vi "SW_Smooth_Image.vi"(6 "Normalize? (F)":bool, 7 "Sigma":dbl=1.0, 8 "Error In":errorcluster, 9 "Image? (T)":bool=TRUE, 10 "Array or pixmap in":u32[][](array[numeric]), 11 "Kernel size":u32=5) -> (0 "Error Out":errorcluster, 3 "Array or pixmap out":u32[][](array[numeric]))   [LabVIEW 2018, in "Tracker.lvlib"]
uses:
  Tracker.lvlib
  <vilib>/Analysis/2dsp.llb/2D Convolution (DBL).vi
  <vilib>/Analysis/NI_AALPro.lvlib
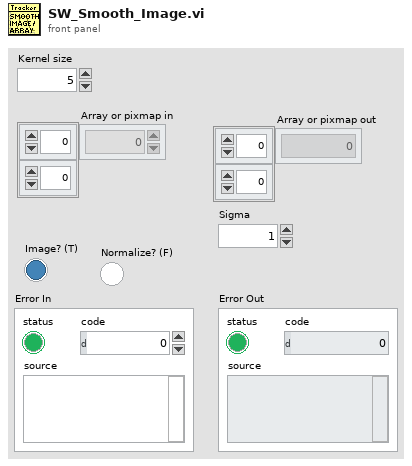
[diagram p1: front panel]
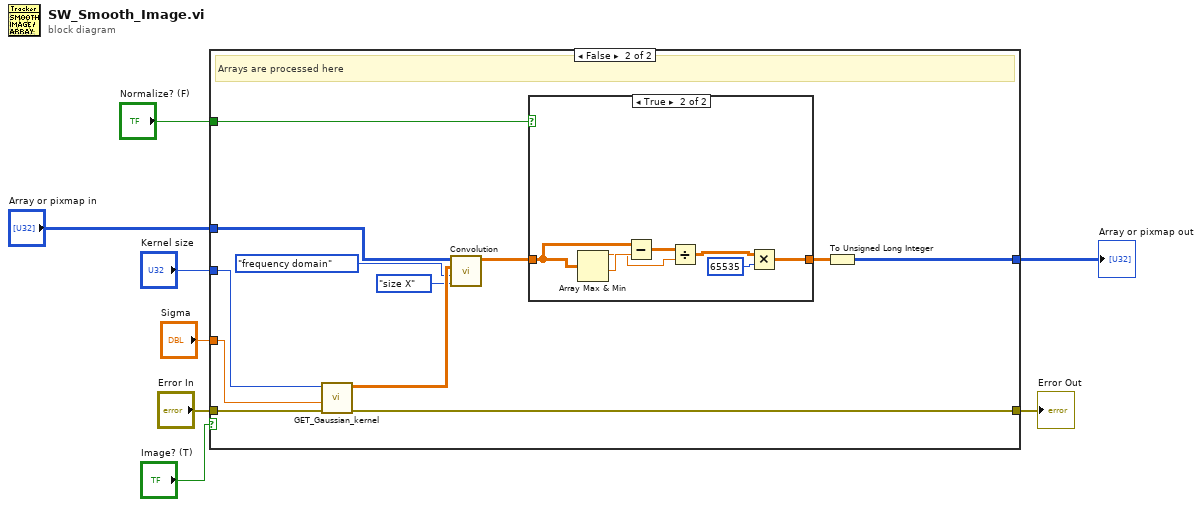
[diagram p0: block diagram]
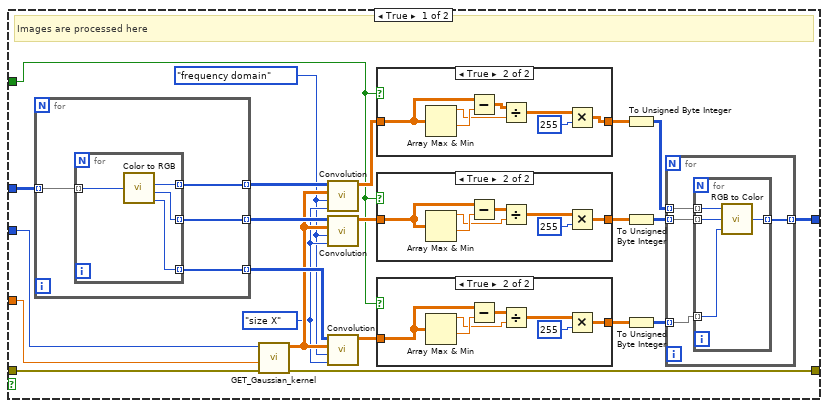
[diagram p2: hidden frame]
diagram:
  n1 = case shown="False" "Image? (T)" {
    tunnel: "Array or pixmap in" -> [w30 w77]
    tunnel: "Kernel size" -> [w29 w82]
    tunnel: "Sigma" -> [w28 w81]
    tunnel: [w18 w74] -> w4
    tunnel: "Error In" -> [w17 w76]
    tunnel: [w16 w75] -> w2
    tunnel: "Normalize? (F)" -> [w10 w71]
    frame True {
      w23 = enum32{"full", "size X", "compact"}."size X" ("output size")
      w22 = enum32{"direct", "frequency domain"}."frequency domain" ("algorithm")
      # "Images are processed here"
      n2 = for {
        tunnel: w30 -> [w66] mode=indexing
        tunnel: [w65] -> w27 mode=indexing
        tunnel: [w64] -> w26 mode=indexing
        tunnel: [w63] -> w25 mode=indexing
        n3 = for {
          tunnel: w66 -> [w70] mode=indexing
          tunnel: [w69] -> w65 mode=indexing
          tunnel: [w68] -> w64 mode=indexing
          tunnel: [w67] -> w63 mode=indexing
          n4 = call <vilib>:"Color to RGB.vi"("Color"=w70) -> ("R"=w69:u8, "G"=w68:u8, "B"=w67:u8)  [unwired: 1 out]
        }
      }
      n5 = call "GET_Gaussian_kernel.vi"("Error In"=w17, "Sigma"=w28, "Kernel size"=w29) -> ("Error Out"=w16:errorcluster, "Gaussian kernel (normalized)"=w24:dbl[][])  [unwired: 7 in]
      n6 = call-poly <vilib>:"Convolution.vi"("output size"=w23, "algorithm"=w22, "Y"=w24, "X"=w27) -> ("X * Y"=w15:dbl[][])  [unwired: 6 in, 1 out]
      n7 = call-poly <vilib>:"Convolution.vi"("output size"=w23, "algorithm"=w22, "Y"=w24, "X"=w26) -> ("X * Y"=w13:dbl[][])  [unwired: 6 in, 1 out]
      n8 = call-poly <vilib>:"Convolution.vi"("output size"=w23, "algorithm"=w22, "Y"=w24, "X"=w25) -> ("X * Y"=w11:dbl[][])  [unwired: 6 in, 1 out]
      n9 = case shown="True" w10 {
        tunnel: w15 -> [w47 w54]
        tunnel: [w47 w48] -> w14
        frame False {
        }
        frame True {
          n10 = Array Max & Min(array=w54) -> (max value=w51:dbl, min value=w53:dbl)  [unwired: 2 out]
          n11 = Subtract(x=w54, y=w53) -> (x-y=w52:dbl[][])
          n12 = Divide(x=w52, y=w51) -> (x/y=w50:dbl[][])
          n13 = Multiply(x=w50, y=255) -> (x*y=w48:dbl[][])
        }
      }
      n14 = case shown="True" w10 {
        tunnel: w13 -> [w39 w46]
        tunnel: [w39 w40] -> w12
        frame False {
        }
        frame True {
          n15 = Array Max & Min(array=w46) -> (max value=w43:dbl, min value=w45:dbl)  [unwired: 2 out]
          n16 = Subtract(x=w46, y=w45) -> (x-y=w44:dbl[][])
          n17 = Divide(x=w44, y=w43) -> (x/y=w42:dbl[][])
          n18 = Multiply(x=w42, y=255) -> (x*y=w40:dbl[][])
        }
      }
      n19 = case shown="True" w10 {
        tunnel: w11 -> [w31 w38]
        tunnel: [w31 w32] -> w9
        frame False {
        }
        frame True {
          n20 = Array Max & Min(array=w38) -> (max value=w35:dbl, min value=w37:dbl)  [unwired: 2 out]
          n21 = Subtract(x=w38, y=w37) -> (x-y=w36:dbl[][])
          n22 = Divide(x=w36, y=w35) -> (x/y=w34:dbl[][])
          n23 = Multiply(x=w34, y=255) -> (x*y=w32:dbl[][])
        }
      }
      n24 = To Unsigned Byte Integer(number=w14) -> (unsigned 8bit integer=w21:u8[][])
      n25 = To Unsigned Byte Integer(number=w12) -> (unsigned 8bit integer=w20:u8[][])
      n26 = To Unsigned Byte Integer(number=w9) -> (unsigned 8bit integer=w19:u8[][])
      n27 = for {
        tunnel: w21 -> [w58] mode=indexing
        tunnel: w20 -> [w57] mode=indexing
        tunnel: w19 -> [w56] mode=indexing
        tunnel: [w55] -> w18 mode=indexing
        n28 = for {
          tunnel: w58 -> [w62] mode=indexing
          tunnel: w57 -> [w61] mode=indexing
          tunnel: w56 -> [w60] mode=indexing
          tunnel: [w59] -> w55 mode=indexing
          n29 = call <vilib>:"RGB to Color.vi"("B"=w60, "G"=w61, "R"=w62) -> ("Color"=w59:u32)
        }
      }
    }
    frame False {
      # "Arrays are processed here"
      n30 = call "GET_Gaussian_kernel.vi"("Error In"=w76, "Sigma"=w81, "Kernel size"=w82) -> ("Error Out"=w75:errorcluster, "Gaussian kernel (normalized)"=w80:dbl[][])  [unwired: 7 in]
      n31 = call-poly <vilib>:"Convolution.vi"("output size"=enum32{"full", "size X", "compact"}."size X", "algorithm"=enum32{"direct", "frequency domain"}."frequency domain", "Y"=w80, "X"=w77) -> ("X * Y"=w73:dbl[][])  [unwired: 6 in, 1 out]
      n32 = case shown="True" w71 {
        tunnel: w73 -> [w83 w90]
        tunnel: [w83 w84] -> w72
        frame False {
        }
        frame True {
          n33 = Array Max & Min(array=w90) -> (max value=w87:dbl, min value=w89:dbl)  [unwired: 2 out]
          n34 = Subtract(x=w90, y=w89) -> (x-y=w88:dbl[][])
          n35 = Divide(x=w88, y=w87) -> (x/y=w86:dbl[][])
          n36 = Multiply(x=w86, y=65535) -> (x*y=w84:dbl[][])
        }
      }
      n37 = To Unsigned Long Integer(number=w72) -> (unsigned 32bit integer=w74:u32[][])
    }
  }
  "Array or pixmap out" <- w4
  "Error Out" <- w2
